vi "SendPPMSCommand.vi"(9 "PpmsCommand":string, 10 "error in (no error)":errorcluster, 11 "Instrument Ref In":refnum<k24>) -> (0 "SendPPMSCommand Error":i32, 1 "PpmsReply":string, 2 "error out":errorcluster, 3 "Instrument Ref Out":refnum<k24>, 4 "ErrorReply":string)   [LabVIEW 2016]
uses:
  C:/user/patrick/hg/levylab_inst_ppms2/lvsrc/PPMS/lvsrc/QDInstrument_LabView/QDInstrument.dll
  QDInstrument.dll
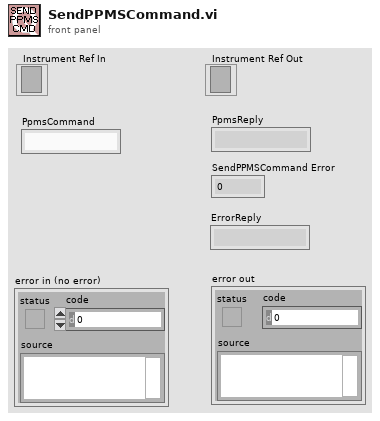
[diagram p1: front panel]
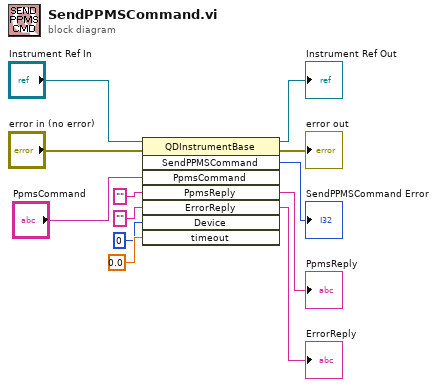
[diagram p0: block diagram]
diagram:
  n1 = invoke class="QDInstrumentBase" method="SendPPMSCommand"(reference="Instrument Ref In", error in="error in (no error)", "PpmsCommand"="PpmsCommand", "PpmsReply"="", "ErrorReply"="", "Device"=0, "timeout"=0.0 ("Result")) -> (reference out=→"Instrument Ref Out":refnum<k24>, error out=→"error out":errorcluster, "SendPPMSCommand"=→"SendPPMSCommand Error":i32, "PpmsReply"=→"PpmsReply":string, "ErrorReply"=→"ErrorReply":string)  [unwired: 1 in, 3 out]
